vi "Actor Core.vi"(8 "error in":errorcluster, 11 "Nested in":refnum<class "DemoCameraController.lvclass">) -> (0 "error out":errorcluster, 3 "Actor out":refnum<class "Actor.lvclass">)   [LabVIEW 2020, in "DemoCameraController.lvlib" / "DemoCameraController.lvclass"]
doc: "(<B>Filename</B>: Actor Framework.lvlib:Actor.lvclass:Actor Core.vi)\n\nReceives messages to the actor, reacts to them, and initiates any error handling that may shut the actor down.\n\nDescendant classes may override this VI to append parallel tasks for the actor to complete while it handles messages. Overrides use the Call Parent Method node."
uses:
  DemoCameraController.lvclass
  C:/Program Files/National Instruments/LabVIEW 2020/vi.lib/ActorFramework/Actor/Actor.lvclass
  <vilib>/ActorFramework/Actor/Actor.lvclass
  DemoCameraController.lvclass/DemoCameraController.ctl
  <vilib>/ActorFramework/Actor/Actor.lvclass/Actor.ctl
  <vilib>/ActorFramework/Message Enqueuer/Message Enqueuer.lvclass/Message Enqueuer.ctl
  Model/Hardware Abstraction Layer/Component/Device/Device/DataExchange.ctl
  Model/Hardware Abstraction Layer/Component/Device/Device Messages/StartSequenceAcquisition Msg/StartSequenceAcquisition Msg.lvclass/StartSequenceAcquisition Msg.ctl
  <vilib>/ActorFramework/Message Enqueuer/Init from Existing Queue.vi
  <vilib>/ActorFramework/Message Enqueuer/Enqueue.vi
  Model/Hardware Abstraction Layer/Component/Device/Device Messages/StartSequenceAcquisition Msg/StartSequenceAcquisition Msg.lvclass
  C:/Program Files/National Instruments/LabVIEW 2020/vi.lib/ActorFramework/Message/Message.lvclass
  Model/Hardware Abstraction Layer/Component/Device/Device Messages/StopAcquisition Msg/StopAcquisition Msg.lvclass
  <vilib>/ActorFramework/Stop Msg/Stop Msg.lvclass
  <vilib>/ActorFramework/Message Priority Queue/Priority Enqueue.vi
  <vilib>/ActorFramework/Message Enqueuer/Message Enqueuer.lvclass
  Interface/DataListener/DataListener.lvclass
  Model/Hardware Abstraction Layer/Component/Camera/Camera Messages/SetExposure Msg/SetExposure Msg.lvclass
panel:
  in  "Save Path":path
  in  "Interval":dbl min=0.0 max=99999.0
  in  "Frames":dbl min=0.0 max=5000.0
  in  "ExposureMs":dbl min=0.0 max=99999.0
  in  "Snap":bool
  in  "Live":bool
  in  "Acquire":bool
  in  "Stop":bool
  in  "Album":bool
  in  "Exit":bool
  in  "FrameIndexSroll":i32(c297)
  out "RawImage":T1(plugin-control)
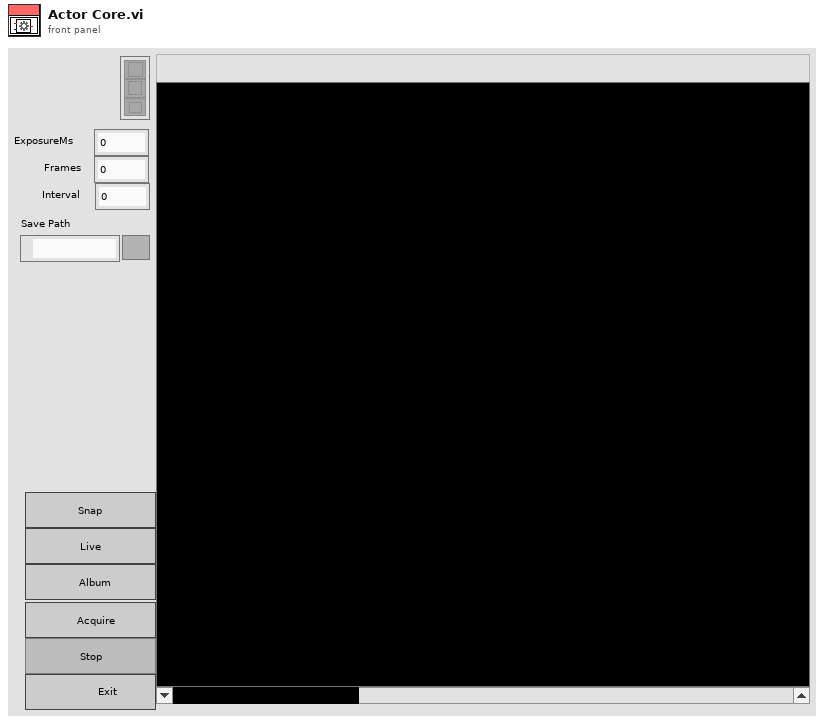
[diagram p1: front panel]
types:
  T1 = typedef "IMAQ Image.ctl" = refnum<image>
  T2 = cluster{"Stop":refnum<user-event>, "RawImage":refnum<user-event>}
  T3 = typedef "DataListener.lvclass/DataExchange.ctl" = cluster{"Source":string, "Target":string, "Type":string, "value":variant}
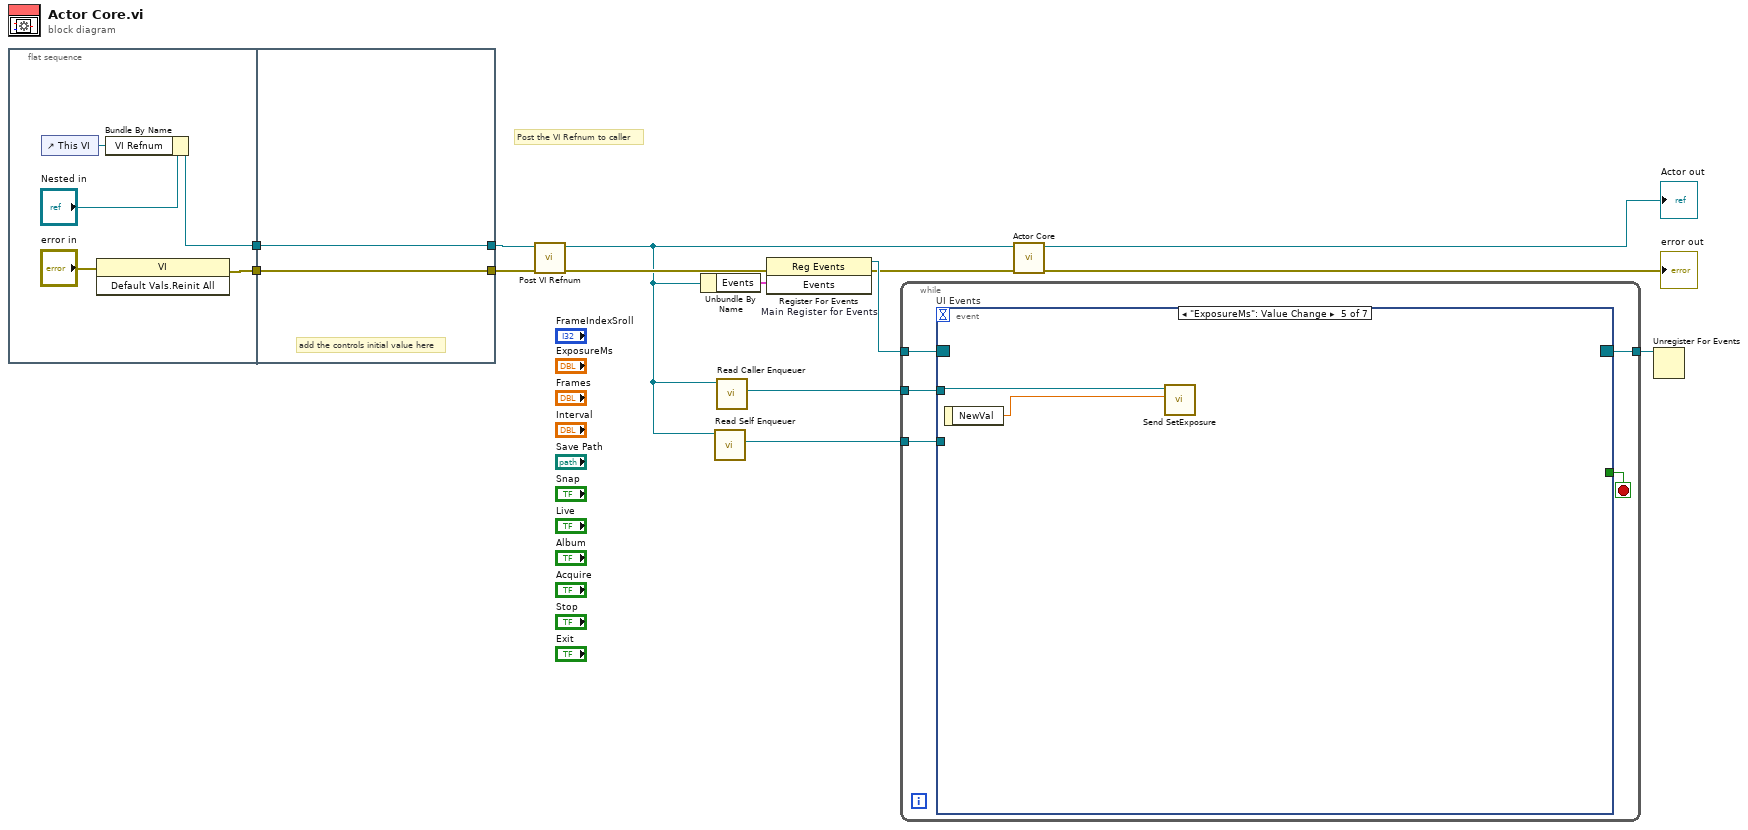
[diagram p0: block diagram]
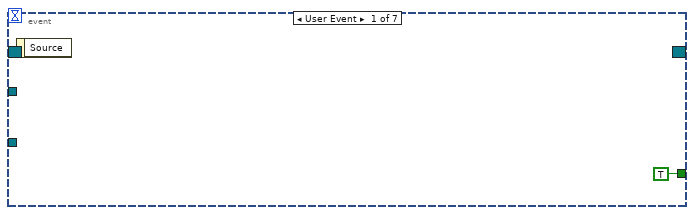
[diagram p2: hidden frame]
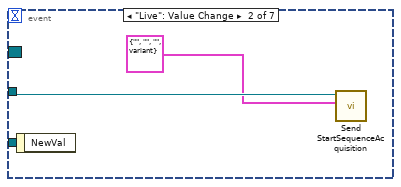
[diagram p3: hidden frame]
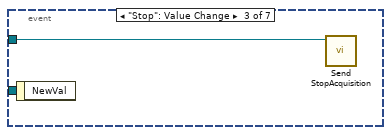
[diagram p4: hidden frame]
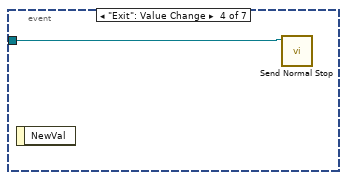
[diagram p5: hidden frame]
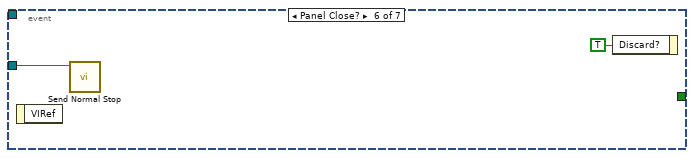
[diagram p6: hidden frame]
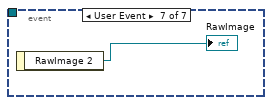
[diagram p7: hidden frame]
diagram:
  # "Post the VI Refnum to caller"
  n1 = flat-sequence {
    tunnel: [w17] -> w6
    tunnel: [w16] -> w5
    tunnel: [w20] -> w3
    tunnel: [w21] -> w7
    tunnel: w6 -> [w21]
    tunnel: w5 -> [w20]
    frame #0 {
      n2 = control-ref of="This VI"() -> (w15:refnum<vi>)
      n3 = invoke class="VI" method="Default Vals.Reinit All"(error in="error in") -> (error out=w17:errorcluster)  [unwired: 2 in, 2 out]
      n4 = Bundle By Name(cluster="Nested in", "VI Refnum"=w15) -> (w16:refnum<class "DemoCameraController.lvclass">)
    }
    frame #1 {
      # "add the controls initial value here"
    }
  }
  n5 = call-dynamic "Post VI Refnum.vi"("error in (no error)"=w7, "Controller Template in"=w3) -> ("error out"=w4:errorcluster, "Controller Template out"=w2:refnum<class "DemoCameraController.lvclass">)  [unwired: 8 in]
  n6 = Unbundle By Name(w2) -> ("Events"=w11:T2)
  n7 = call <vilib>:"Read Self Enqueuer.vi"("Actor"=w2) -> ("Self Enqueuer"=w9:refnum<class "Message Enqueuer.lvclass">)  [unwired: 10 in]
  n8 = call <vilib>:"Read Caller Enqueuer.vi"("Actor"=w2) -> ("Caller Enqueuer"=w1:refnum<class "Message Enqueuer.lvclass">)  [unwired: 10 in]
  n9 = register-events "Main Register for Events"(error in=w4, w11) -> (reference out=w12:refnum<event-registration>, error out=w8:errorcluster)  [unwired: 1 in]
  n10 = while {
    tunnel: w12 -> [w26]
    tunnel: [w24] -> w10
    tunnel: w9 -> [w23]
    tunnel: w1 -> [w22]
    stop <- w25 stop-if-true
    n11 = event "UI Events" shown="[4] \"ExposureMs\": Value Change" {
      selector: w26 -> [_ _ _ _ _ _ _]
      dyn-events: [_ _ _ _ _ _ _] -> w24
      timeout: _ -> [_ _ _ _ _ _ _]
      tunnel: [TRUE _ _ _ _ _ _] -> w25
      tunnel: w23 -> [_ _ _ w31 _ w34 _]
      tunnel: w22 -> [_ w29 w30 _ w33 _ _]
      event User Event {
        n12 = event-data() -> ()  [unwired: 1 in, 1 out]
      }
      event "Live": Value Change {
        n13 = event-data() -> ()  [unwired: 1 in, 1 out]
        n14 = call "Send StartSequenceAcquisition.vi"("DataExchange"=T3 {"Source"="", "Target"="", "Type"="", "value"=variant}, "Message Enqueuer"=w29) -> ()  [unwired: 8 in, 2 out]
      }
      event "Stop": Value Change {
        n15 = event-data() -> ()  [unwired: 1 in, 1 out]
        n16 = call "Send StopAcquisition.vi"("Message Enqueuer"=w30) -> ()  [unwired: 9 in, 2 out]
      }
      event "Exit": Value Change {
        n17 = event-data() -> ()  [unwired: 1 in, 1 out]
        n18 = call <vilib>:"Send Normal Stop.vi"("Message Enqueuer"=w31) -> ()  [unwired: 10 in, 1 out]
      }
      event "ExposureMs": Value Change {
        n19 = event-data() -> ("NewVal"=w32:dbl)  [unwired: 1 in]
        n20 = call "Send SetExposure.vi"("Setting.Exposure"=w32, "Message Enqueuer"=w33) -> ()  [unwired: 8 in, 2 out]
      }
      event Panel Close? {
        n21 = event-data() -> ()  [unwired: 1 in, 1 out]
        n22 = call <vilib>:"Send Normal Stop.vi"("Message Enqueuer"=w34) -> ()  [unwired: 10 in, 1 out]
        n23 = event-data("Discard?"=TRUE) -> ()  [unwired: 1 in, 1 out]
      }
      event User Event {
        n24 = event-data() -> ("RawImage 2"=→"RawImage":T1)  [unwired: 1 in]
      }
    }
  }
  n25 = call-parent "Actor Core.vi"("error in"=w8, "Actor in"=w2) -> ("error out"=→"error out":errorcluster, "Actor out"=→"Actor out":refnum<class "Actor.lvclass">)  [unwired: 8 in]
  n26 = Unregister For Events(event registration refnum=w10) -> ()  [unwired: 1 in, 1 out]
